vi "Read Init VI.vi"(8 "error in":errorcluster, 11 "Custom Device reference in":refnum<k24>) -> (0 "error out":errorcluster caption="error in", 2 "Initialization VI":T1={"Execution"=enum."silent", "Path"={"Path"=path "", "Path Type"=enum."Absolute"}, "Type"=enum."VI", "Position"=enum."centered"}, 3 "Custom Device reference out":refnum<k24>)   [LabVIEW 2015, in "Configuration Tool.lvlib"]
uses:
  Configuration Tool.lvlib
  NationalInstruments.VeriStand.XMLReader
  XML Controls/Initialization VI.ctl
  XML Controls/Execution Types.ctl
  XML Controls/Path Cluster.ctl
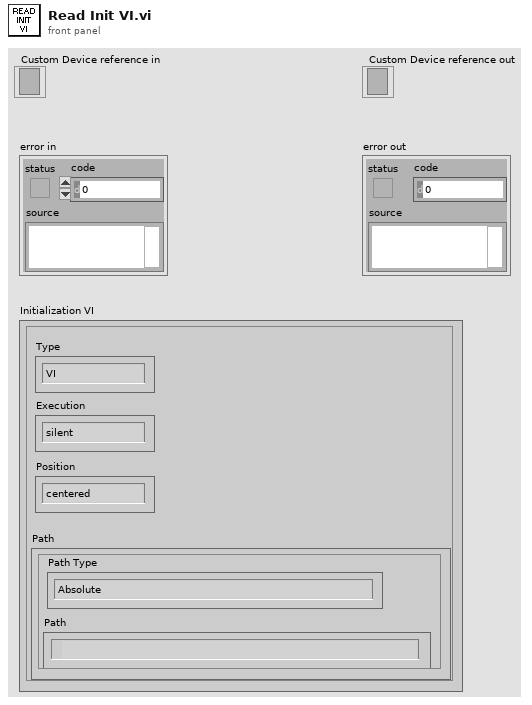
[diagram p1: front panel]
types:
  T1 = typedef "Configuration Tool.lvlib/Initialization VI.ctl" = cluster{"Execution":T2, "Path":T3, "Type":enum16{"Action", "VI"}, "Position":enum16{"centered", "mouse pointer"}}
  T2 = typedef "Configuration Tool.lvlib/Execution Types.ctl" = enum16{"silent", "modal", "floating", "default"}
  T3 = typedef "Configuration Tool.lvlib/Path Cluster.ctl" = cluster{"Path":path, "Path Type":enum16{"Absolute", "To Base", "To Common Doc Dir", "To Application Data Dir"}}
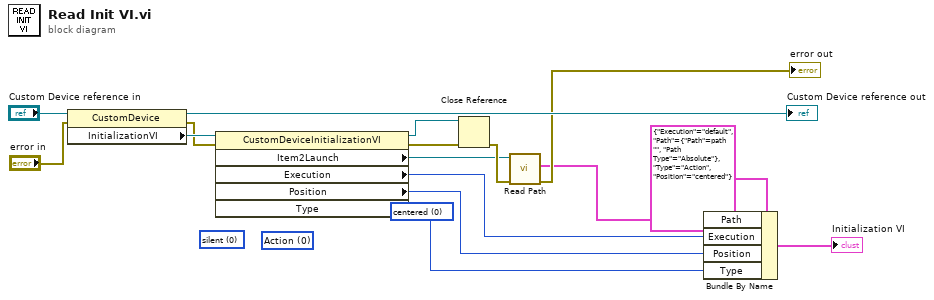
[diagram p0: block diagram]
diagram:
  (unwired) 0 items=["centered", "mousepointer"] ("Position")
  (unwired) 0 items=["Action", "VI"] ("Type")
  (unwired) 0 items=["silent", "modal", "floating", "default"] ("Execution")
  n1 = property class="CustomDevice"(reference="Custom Device reference in", error in="error in") -> (reference out=→"Custom Device reference out":refnum<k24>, error out=w13:errorcluster, "InitializationVI"=w14:refnum<k24>)
  n2 = property class="CustomDeviceInitializationVI"(reference=w14, error in=w13) -> (reference out=w10:refnum<k24>, error out=w9:errorcluster, "Item2Launch"=w5:refnum<k24>, "Execution"=w3:i32, "Position"=w2:i32, "Type"=w1:i32)
  n3 = Close Reference(reference=w10, error in (no error)=w9) -> (error out=w8:errorcluster)
  n4 = call "Read Path.vi"("error in (no error)"=w8, "Path Ref"=w5) -> ("error out"=→"error out":errorcluster, "Path"=w4:T3)  [unwired: 8 in]
  n5 = Bundle By Name(cluster=T1 {"Execution"=enum."default", "Path"={"Path"=path "", "Path Type"=enum."Absolute"}, "Type"=enum."Action", "Position"=enum."centered"} ("Initialization VI"), "Path"=w4, "Execution"=w3, "Position"=w2, "Type"=w1) -> (→"Initialization VI":T1)
